vi "SetTripPoint00.vi"() -> ()   [LabVIEW 2011]
panel:
  out "concatenated string":string
  in  "point":dbl=1.0 min=1.0 max=2.0 step=1.0 format="%#_1g"
  in  "Trip Point (Torr)":dbl=700.0
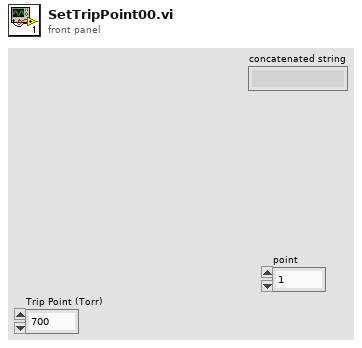
[diagram p1: front panel]
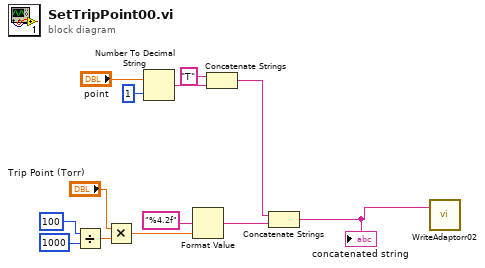
[diagram p0: block diagram]
diagram:
  n1 = Divide(x=100, y=1000) -> (x/y=w11:dbl)
  n2 = Multiply(x="Trip Point (Torr)", y=w11) -> (x*y=w7:dbl)
  n3 = Number To Decimal String(number="point", width (-)=i16 1) -> (decimal integer string=w3:string)
  n4 = Format Value(format string="%4.2f", value (0)=w7) -> (output string=w9:string)  [unwired: 1 in]
  n5 = Concatenate Strings("T" ("string"), w3) -> (w1:string)
  n6 = Concatenate Strings(w1, w9) -> (w8:string)
  "concatenated string" <- w8
  n7 = call "WriteAdaptorr02.vi"("string to write"=w8) -> ()  [unwired: 1 in, 1 out]
